vi "Is a Number.vi"(1 "string":string) -> (0 "is a number?":bool)   [LabVIEW 2025]
uses:
  <vilib>/Utility/error.llb/Trim Whitespace One-Sided.vi
  <vilib>/regexp/Match Regular Expression.xnode
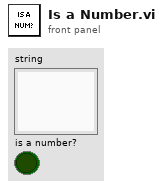
[diagram p1: front panel]
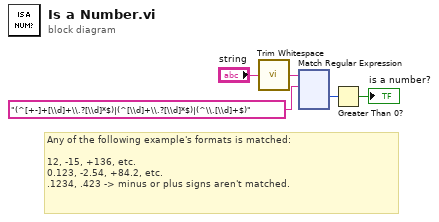
[diagram p0: block diagram]
diagram:
  # "Any of the following example's formats is matched:\n\n12, -15, +136, etc.\n0.123, -2.54, +84.2, etc.\n.1234, .423 -> minus or plus signs aren't matched."
  n1 = call <vilib>:"Trim Whitespace.vi"("string"="string") -> ("trimmed string"=w5:string)  [unwired: 1 in]
  n2 = xnode "Match Regular Expression"("input string"=w5, "regular expression"="(^[+-]+[\\d]+\\.?[\\d]*$)|(^[\\d]+\\.?[\\d]*$)|(^\\.[\\d]+$)") -> ("offset past match"=w4:i32)  [unwired: 4 in, 4 out]
  n3 = Greater Than 0?(x=w4) -> (x > 0?=→"is a number?":bool)
